vi "2 计算x阶层和.vi"() -> ()   [LabVIEW 2019]
panel:
  out "y":i32
  in  "x":i32
  out "x阶层":i32
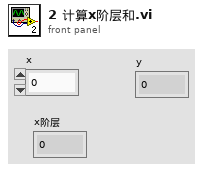
[diagram p1: front panel]
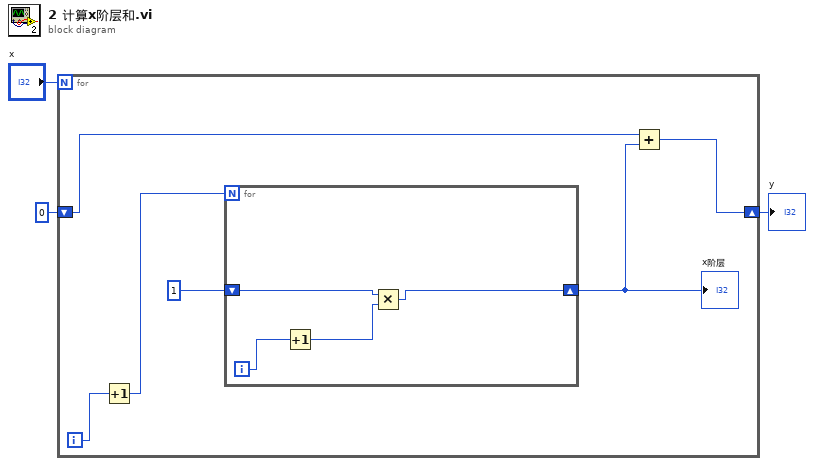
[diagram p0: block diagram]
diagram:
  n1 = for {
    N: "x" -> [_]
    shift-right: [w4] -> w1
    shift-left: 0 -> [w6]
    i -> [w8]
    n2 = Increment(x=w8) -> (x+1=w7:i32)
    n3 = for {
      N: w7 -> [_]
      shift-right: [w10] -> w5
      shift-left: 1 -> [w11]
      i -> [w13]
      n4 = Increment(x=w13) -> (x+1=w12:i32)
      n5 = Multiply(x=w11, y=w12) -> (x*y=w10:i32)
    }
    "x阶层" <- w5
    n6 = Add(x=w6, y=w5) -> (x+y=w4:i32)
  }
  "y" <- w1
